vi "Format Read Command.vi"(4 "error in":errorcluster, 5 "Variable to Read":T1, 6 "Flow Meter DevID":i32=1, 7 "VISA resource name":refnum<visa-resource-name>) -> (0 "error out":errorcluster, 1 "Length Bytes (Dec)":i32, 2 "Command String with Checksum":string, 3 "VISA resource name out":refnum<visa-resource-name>)   [LabVIEW 2010, in "FEM-03.lvlib"]
uses:
  Controls/Variable List.ctl
  FEM-03.lvlib
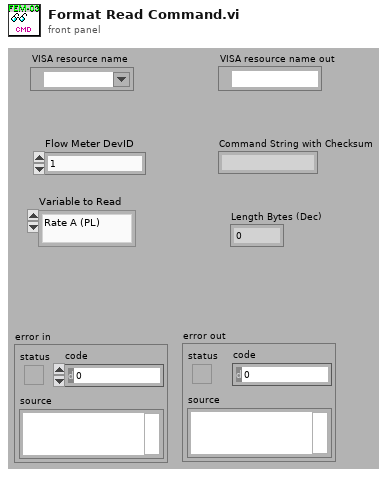
[diagram p1: front panel]
types:
  T1 = typedef "FEM-03.lvlib/Variable List.ctl" = enum16{"Rate A (PL)", "Rate A (GT)", "Job Total A", "Grand Total A", "A-KFR for Rate", "A-KFR decimal point location", "A-KFT for Total", "A-KFT decimal point location ", "A-Rate Engineering Units", "A-Total Engineering units", "A-Flow Direction", "Rate B (PL)", "Rate B (GT)", "Job Total B", "Grand Total B", "B-KFR for Rate", "B-KFR deciminal point location", "B-Rate Engineering units", "B-KFT for Total", "B-KFT decimal point location", "B-Total Engineering units", "Limit 1 Mode", "Limit1", "Margin 1 for rate limit", "Limit 2 Mode", "Limit2", "Margin 2 for rate limit", "Milli-amps Offset", "Milli-amps Out", "Analog Out Mode", "Serial Speed", "Unit Number", "Serial RESET TOTAL", "Update EEPROM", "Relay Override", "FORCE mA Output"}
  T2 = typedef "FEM-03.lvlib/Variable Info.ctl" = cluster{"Hex Address (String)":string, "Length Bytes (String)":string, "Length Bytes (Dec)":i32, "Multibyte format":enum16{"MSB First", "Array last digit 0", "None"}}
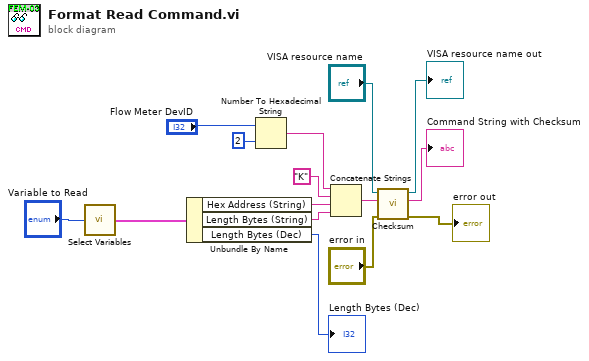
[diagram p0: block diagram]
diagram:
  n1 = call "Select Variables.vi"("Variables"="Variable to Read") -> ("Variable Info"=w7:T2)
  n2 = Unbundle By Name(w7) -> ("Hex Address (String)"=w5:string, "Length Bytes (String)"=w6:string, "Length Bytes (Dec)"=→"Length Bytes (Dec)":i32)
  n3 = Number To Hexadecimal String(1:i16 2 ("width (-)"), 2:"Flow Meter DevID") -> (0:w3:string)
  n4 = Concatenate Strings(w3, "K" ("string"), w5, w6) -> (w8:string)
  n5 = call "Checksum.vi"("error in"="error in", "Command String"=w8, "VISA resource name"="VISA resource name") -> ("error out"=→"error out":errorcluster, "Command String with Checksum"=→"Command String with Checksum":string, "VISA resource name out"=→"VISA resource name out":refnum<visa-resource-name>)  [unwired: 5 in, 1 out]
